vi "Programmatic SV Creation.vi"() -> ()   [LabVIEW 2014]
panel:
  in  "Name of new library":string="New Library.lvlib"
  out "error out":errorcluster
  in  "Project Path":path=path "C:/Programmatic SV Creation.lvproj"
  # "Instructions:\n1. Browse to the path where you saved the .lvproj LabVIEW Project.\n2. Run the VI."
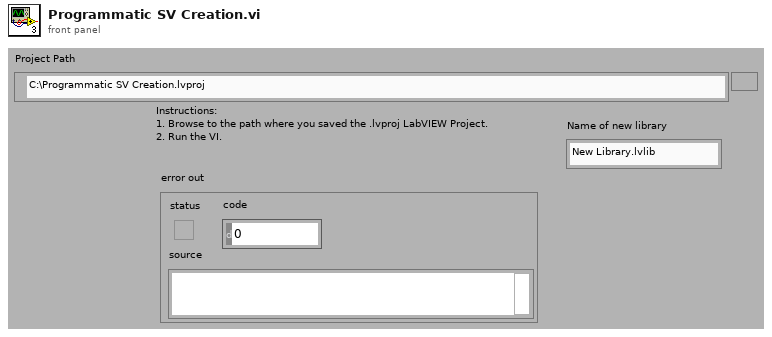
[diagram p1: front panel]
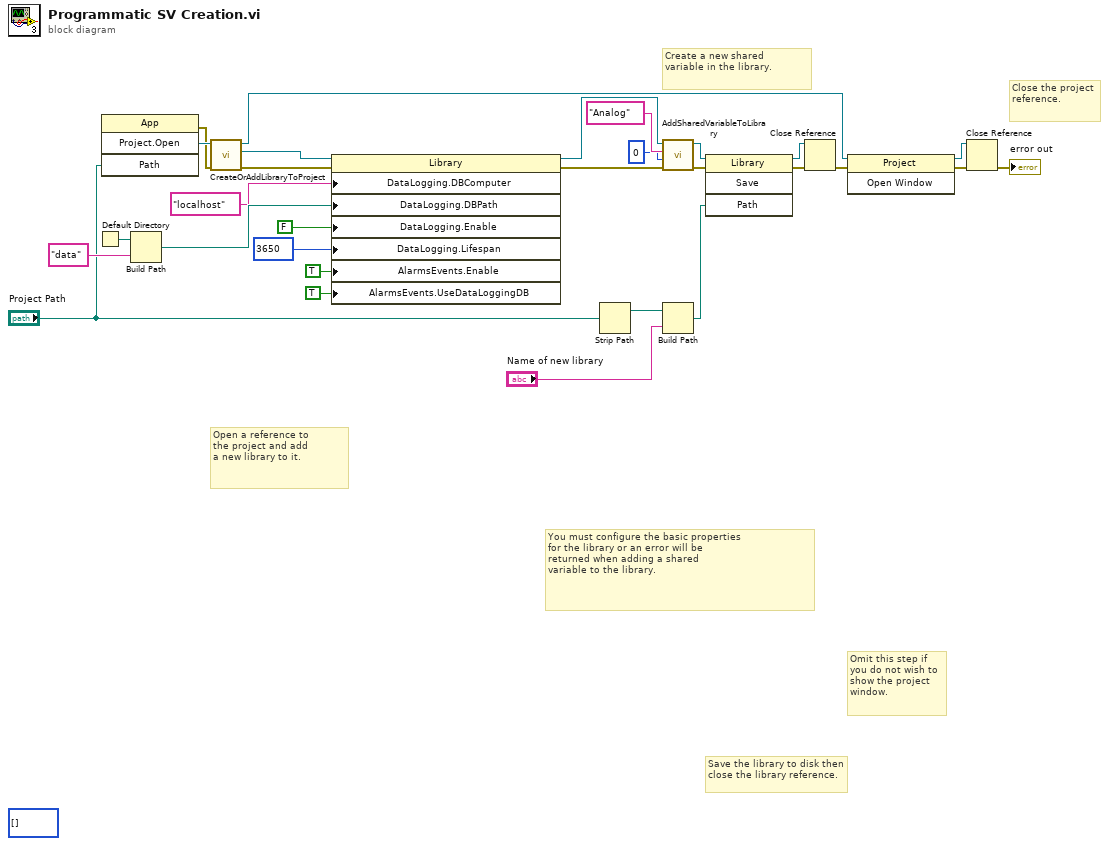
[diagram p0: block diagram]
diagram:
  (unwired) i32[] []
  # "Create a new shared\nvariable in the library."
  # "You must configure the basic properties\nfor the library or an error will be\nreturned when adding a shared\nvariable to the library."
  # "Open a reference to\nthe project and add\na new library to it."
  # "Close the project reference."
  # "Omit this step if you do not wish to show the project window."
  # "Save the library to disk then close the library reference."
  n1 = Default Directory() -> (w27:path)
  n2 = invoke class="App" method="Project.Open"("Path"="Project Path") -> (error out=w20:errorcluster, "Project:Open"=w21:refnum<vi>)  [unwired: 3 in, 2 out]
  n3 = Build Path(base path=w27, name or relative path="data") -> (appended path=w29:path)
  n4 = call <vilib>:"CreateOrAddLibraryToProject.vi"("error in (no error)"=w20, "Project Reference In (Create New)"=w21) -> ("error out"=w18:errorcluster, "Library Reference Out"=w19:refnum<vi>, "Project Reference Out"=w6:refnum<vi>)  [unwired: 7 in]
  n5 = property class="Library"(reference=w19, error in=w18, "DataLogging.DBComputer"="localhost" ("AlarmsEvents:Database Computer"), "DataLogging.DBPath"=w29, "DataLogging.Enable"=FALSE ("DataLogging:Enable"), "DataLogging.Lifespan"=u32 3650 ("DataLogging:Lifespan"), "AlarmsEvents.Enable"=TRUE ("AlarmsEvents:Enable"), "AlarmsEvents.UseDataLoggingDB"=TRUE ("AlarmsEvents:Use DataLogging Database")) -> (reference out=w10:refnum<vi>, error out=w9:errorcluster)
  n6 = Strip Path(path="Project Path") -> (stripped path=w4:path)  [unwired: 1 out]
  n7 = call <vilib>:"AddSharedVariableToLibrary.vi"("error in (no error)"=w9, "Variable Data Type (Double)"=0, "Variable Name"="Analog", "Library Reference In"=w10) -> ("error out"=w7:errorcluster, "Library Reference Out"=w8:refnum<vi>)  [unwired: 5 in, 1 out]
  n8 = Build Path(base path=w4, name or relative path="Name of new library") -> (appended path=w5:path)
  n9 = invoke class="Library" method="Save"(reference=w8, error in=w7, "Path"=w5) -> (reference out=w17:refnum<vi>, error out=w16:errorcluster)  [unwired: 1 in, 2 out]
  n10 = Close Reference(reference=w17, error in (no error)=w16) -> (error out=w13:errorcluster)
  n11 = invoke class="Project" method="Open Window"(reference=w6, error in=w13) -> (reference out=w14:refnum<vi>, error out=w12:errorcluster)  [unwired: 1 in, 1 out]
  n12 = Close Reference(reference=w14, error in (no error)=w12) -> (error out=→"error out":errorcluster)
